vi "Build Report String.vi"(8 "error in (no error)":errorcluster, 10 "Result":T1, 11 "Mouse Action in":refnum<class "Mouse Action.lvclass">) -> (0 "error out":errorcluster, 2 "Report String":string, 3 "Mouse Action out":refnum<class "Mouse Action.lvclass">)   [LabVIEW 2020, in "MacroAssert.lvlib" / "Mouse Action.lvclass"]
doc: "Builds a string using <B>Step</B> and <B>Result</B> to be included in a report."
uses:
  Mouse Action.lvclass
  CTLs/Result.ctl
  CTLs/Outcome.ctl
  Action Step/Action Step.lvclass
  MacroAssert.lvlib
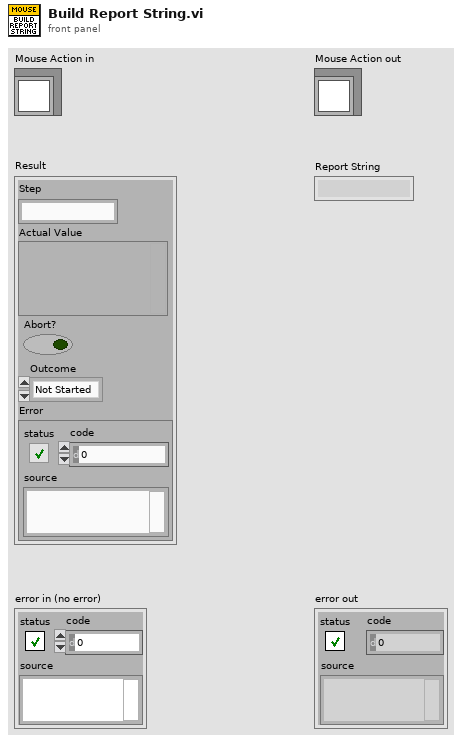
[diagram p1: front panel]
types:
  T1 = typedef "MacroAssert.lvlib/Result.ctl" = cluster{"Step":string, "Actual Value":variant, "Abort?":bool, "Outcome":T2, "Error":errorcluster}
  T2 = typedef "MacroAssert.lvlib/Outcome.ctl" = enum16{"Not Started", "Skipped", "Pass", "Fail", "Complete", "Error", "Auto Abort", "User Abort"}
  T3 = typedef "MacroAssert.lvlib/Mouse Action.lvclass/Mouse Action Type.ctl" = enum16{"Click", "Absolute Move", "Absolute Move and Click", "Relative Move", "Relative Move and Click", "Wheel Up", "Wheel Down"}
  T4 = typedef "MacroAssert.lvlib/Mouse Action.lvclass/Click Type.ctl" = enum16{"Normal", "Hold", "Release"}
  T5 = typedef "MacroAssert.lvlib/Mouse Action.lvclass/Button.ctl" = enum16{"Left", "Right", "Middle"}
  T6 = typedef "MacroAssert.lvlib/Mouse Action.lvclass/Relative Movement Type.ctl" = enum16{"Pixels from Current Position", "Pixels from Top-Left of Control", "Pixels from Top-Left of Window", "Percentage from Top-Left of Control", "Percentage from Top-Left of Window", "Percentage from Top-Left of Screen"}
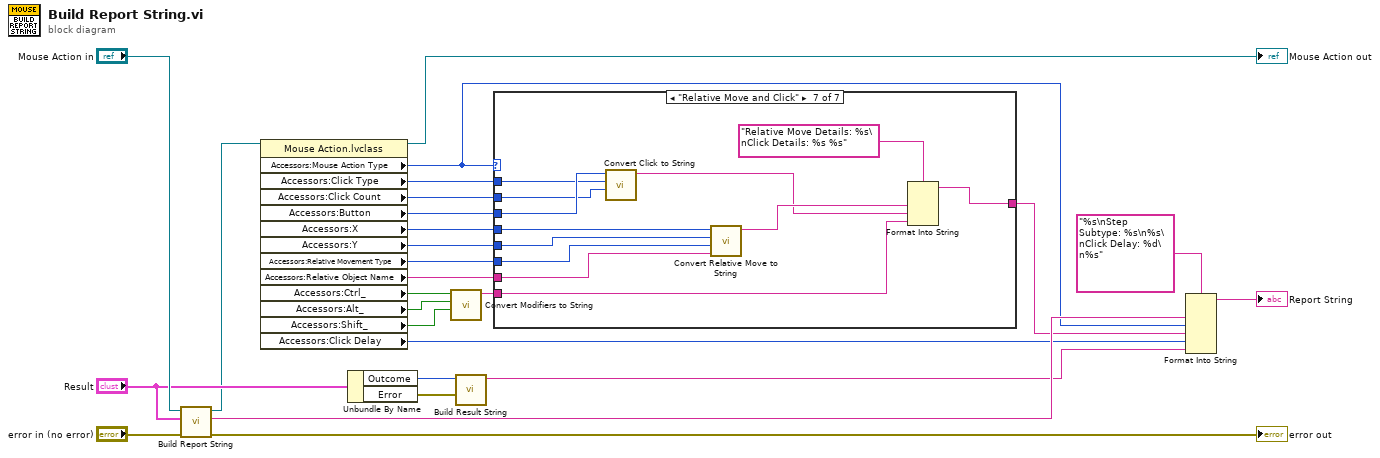
[diagram p0: block diagram]
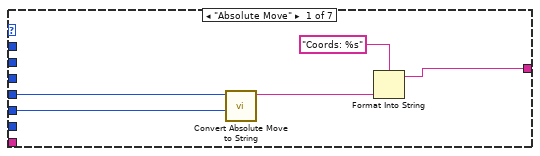
[diagram p2: hidden frame]
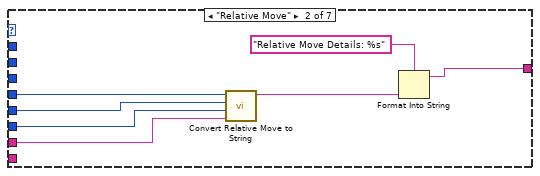
[diagram p3: hidden frame]
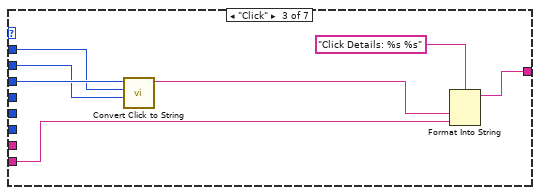
[diagram p4: hidden frame]
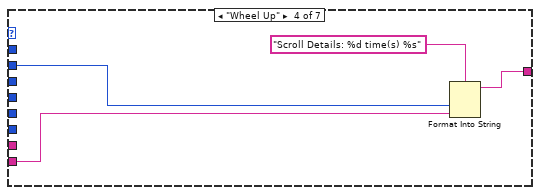
[diagram p5: hidden frame]
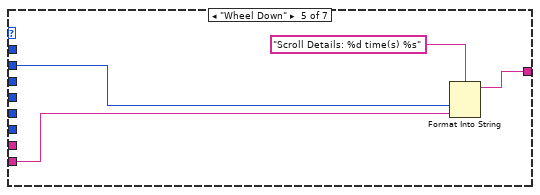
[diagram p6: hidden frame]
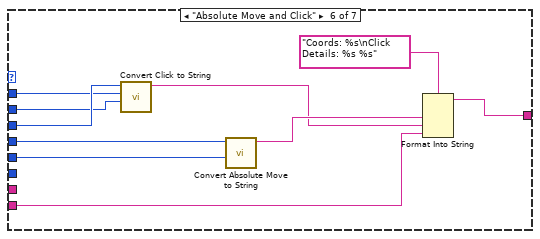
[diagram p7: hidden frame]
diagram:
  n1 = call-parent "Build Report String.vi"("error in (no error)"="error in (no error)", "Result"="Result", "Step in"="Mouse Action in") -> ("error out"=→"error out":errorcluster, "Report String"=w25:string, "Step out"=w6:refnum<class "Mouse Action.lvclass">)  [unwired: 6 in]
  n2 = property class="Mouse Action.lvclass"(reference=w6) -> (reference out=→"Mouse Action out":refnum<class "Mouse Action.lvclass">, "Accessors:Mouse Action Type"=w4:T3, "Accessors:Click Type"=w14:T4, "Accessors:Click Count"=w13:i32, "Accessors:Button"=w15:T5, "Accessors:X"=w17:i32, "Accessors:Y"=w16:i32, "Accessors:Relative Movement Type"=w10:T6, "Accessors:Relative Object Name"=w9:string, "Accessors:Ctrl_"=w12:bool, "Accessors:Alt_"=w8:bool, "Accessors:Shift_"=w11:bool, "Accessors:Click Delay"=w1:i32)  [unwired: 1 in, 1 out]
  n3 = Unbundle By Name("Result") -> ("Outcome"=w24:T2, "Error"=w23:errorcluster)
  n4 = call "Convert Modifiers to String.vi"("Shift?"=w11, "Alt?"=w8, "Ctrl?"=w12) -> ("String"=w7:string)  [unwired: 8 in]
  n5 = call "Build Result String.vi"("Error"=w23, "Outcome"=w24) -> ("Result String"=w2:string)  [unwired: 9 in]
  n6 = case shown="\"Relative Move and Click\"" w4 {
    tunnel: [w27 w32 w44 w48 w52 w54 w68] -> w3
    tunnel: w17 -> [w31 w38 _ _ _ w63 w67]
    tunnel: w16 -> [w30 w37 _ _ _ w62 w66]
    tunnel: w15 -> [_ _ w42 _ _ w58 w72]
    tunnel: w14 -> [_ _ w41 _ _ w57 w71]
    tunnel: w13 -> [_ _ w40 w47 w51 w56 w70]
    tunnel: w7 -> [_ _ w43 w46 w50 w59 w73]
    tunnel: w10 -> [_ w36 _ _ _ _ w65]
    tunnel: w9 -> [_ w35 _ _ _ _ w64]
    frame "Absolute Move" {
      n7 = call "Convert Absolute Move to String.vi"("Y"=w30, "X"=w31) -> ("String"=w28:string)  [unwired: 9 in]
      n8 = Format Into String(format string="Coords: %s", w28) -> (resulting string=w27:string)  [unwired: 2 in, 1 out]
    }
    frame "Relative Move" {
      n9 = call "Convert Relative Move to String.vi"("Relative Object Name"=w35, "Relative Movement Type"=w36, "Y"=w37, "X"=w38) -> ("String"=w33:string)  [unwired: 7 in]
      n10 = Format Into String(format string="Relative Move Details: %s", w33) -> (resulting string=w32:string)  [unwired: 2 in, 1 out]
    }
    frame "Click" {
      n11 = call "Convert Click to String.vi"("Click Count"=w40, "Click Type"=w41, "Button"=w42) -> ("Click String"=w39:string)  [unwired: 8 in]
      n12 = Format Into String(format string="Click Details: %s %s", w39, w43) -> (resulting string=w44:string)  [unwired: 2 in, 1 out]
    }
    frame "Wheel Up" {
      n13 = Format Into String(format string="Scroll Details: %d time(s) %s", w47, w46) -> (resulting string=w48:string)  [unwired: 2 in, 1 out]
    }
    frame "Wheel Down" {
      n14 = Format Into String(format string="Scroll Details: %d time(s) %s", w51, w50) -> (resulting string=w52:string)  [unwired: 2 in, 1 out]
    }
    frame "Absolute Move and Click" {
      n15 = call "Convert Click to String.vi"("Click Count"=w56, "Click Type"=w57, "Button"=w58) -> ("Click String"=w55:string)  [unwired: 8 in]
      n16 = call "Convert Absolute Move to String.vi"("Y"=w62, "X"=w63) -> ("String"=w60:string)  [unwired: 9 in]
      n17 = Format Into String(format string="Coords: %s\nClick Details: %s %s", w60, w55, w59) -> (resulting string=w54:string)  [unwired: 2 in, 1 out]
    }
    frame "Relative Move and Click" {
      n18 = call "Convert Click to String.vi"("Click Count"=w70, "Click Type"=w71, "Button"=w72) -> ("Click String"=w69:string)  [unwired: 8 in]
      n19 = call "Convert Relative Move to String.vi"("Relative Object Name"=w64, "Relative Movement Type"=w65, "Y"=w66, "X"=w67) -> ("String"=w74:string)  [unwired: 7 in]
      n20 = Format Into String(format string="Relative Move Details: %s\nClick Details: %s %s", w74, w69, w73) -> (resulting string=w68:string)  [unwired: 2 in, 1 out]
    }
  }
  n21 = Format Into String(format string="%s\nStep Subtype: %s\n%s\nClick Delay: %d\n%s", w25, w4, w3, w1, w2) -> (resulting string=→"Report String":string)  [unwired: 2 in, 1 out]
